vi "ZMC Down Mem Zar.vi"(7 "pfilenameinControl":string, 8 "error in (no error)":errorcluster caption="错误输入（无错误）", 9 "buffsize":u32, 10 "pbuffer":string, 11 "handle":u32) -> (0 "error out":errorcluster caption="错误输出", 2 "function return":i32, 3 "handle out":u32)   [LabVIEW 2015, in "zauxdll.lvlib"]
doc: "int32 __stdcall ZMC_DownMemZar(ZMC_HANDLE handle, const char* pbuffer, uint32 buffsize, const char* pfilenameinControl);"
uses:
  zauxdll.lvlib
  zmotion.dll
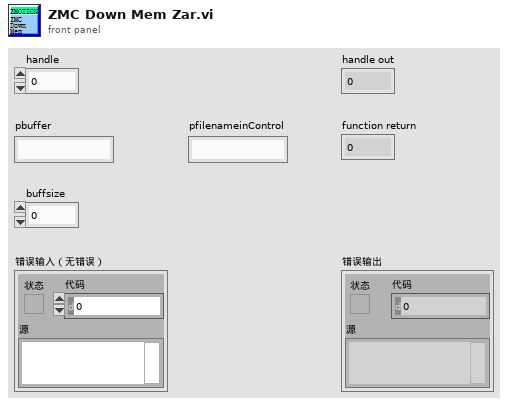
[diagram p1: front panel]
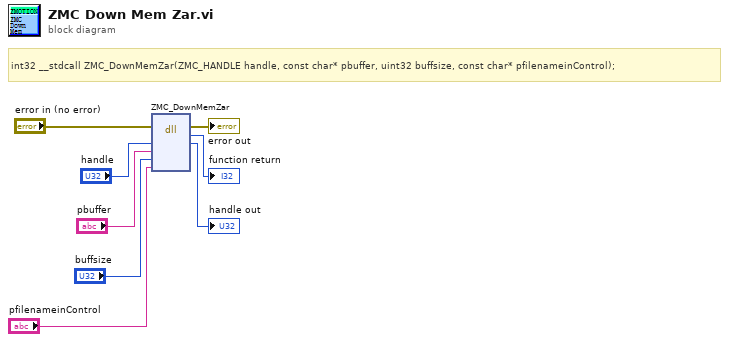
[diagram p0: block diagram]
diagram:
  # "int32 __stdcall ZMC_DownMemZar(ZMC_HANDLE handle, const char* pbuffer, uint32 buffsize, const char* pfilenameinControl);"
  n1 = dll-call lib="C:/Users/VIC/Desktop/GOGORO_SA/system/LLB/zmotion/zaux/zmotion.*" fn="ZMC_DownMemZar"(error in="error in (no error)", "handle"="handle", "pbuffer"="pbuffer", "buffsize"="buffsize", "pfilenameinControl"="pfilenameinControl") -> (error out=→"error out":errorcluster, →"function return":i32, "handle"=→"handle out":u32)  [unwired: 5 in, 1 out]
